vi "AlazarSetRecordSize.vi"(3 "error in (no error)":errorcluster, 4 "Post-trigger Samples":u32, 5 "Pre-trigger Samples":u32, 6 "Handle":u64) -> (0 "error out":errorcluster, 1 "Return Code":u32, 2 "Handle":u64)   [LabVIEW 2023]
doc: "Set the number of pre- and post-trigger samples per record."
uses:
  ATSApi.dll
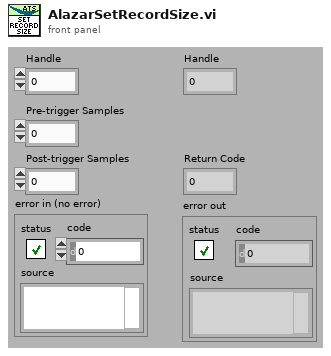
[diagram p1: front panel]
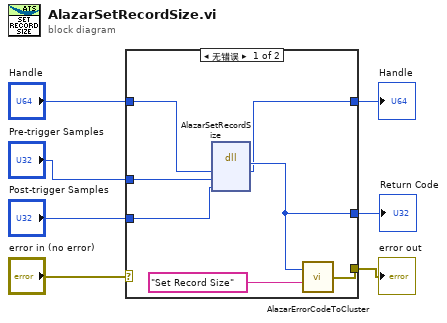
[diagram p0: block diagram]
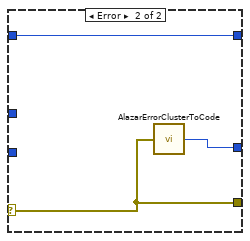
[diagram p2: hidden frame]
diagram:
  n1 = case shown="无错误" "error in (no error)" {
    selector: "error in (no error)" -> [_ w17]
    tunnel: [w11 w17] -> w6
    tunnel: [w13 w16] -> w5
    tunnel: "Handle" -> [w14 w15]
    tunnel: [w10 w15] -> w3
    tunnel: "Pre-trigger Samples" -> [w9 _]
    tunnel: "Post-trigger Samples" -> [w8 _]
    frame No Error {
      n2 = dll-call lib="ATSApi.dll" fn="AlazarSetRecordSize"("handle"=w14, "preTriggerSamples"=w9, "postTriggerSamples"=w8) -> ("return type"=w13:u32, "handle"=w10:u64)  [unwired: 5 in, 2 out]
      n3 = call "AlazarErrorCodeToCluster.vi"("Message"="Set Record Size", "Error Code"=w13) -> ("error out"=w11:errorcluster)
    }
    frame Error {
      n4 = call "AlazarErrorClusterToCode.vi"("error in (no error)"=w17) -> ("Error Code"=w16:u32)
    }
  }
  "Handle" <- w3
  "error out" <- w6
  "Return Code" <- w5
